vi "Query Output Operation Mode.vi"(8 "error in (no error)":errorcluster, 10 "Platform Slot Number (10)":i16=10 min=-1 max=255, 11 "VISA resource name":refnum<visa-resource-name>) -> (0 "error out":errorcluster, 2 "Operation Mode":string, 3 "VISA resource name out":refnum<visa-resource-name>)   [LabVIEW 2018, in "LTB-1.lvlib" / "3150.lvlib"]
doc: "Queries the current operation mode (ABSolute|XB|REFerence) for the active control mode (ATTenuation or POWer)."
uses:
  3150.lvlib
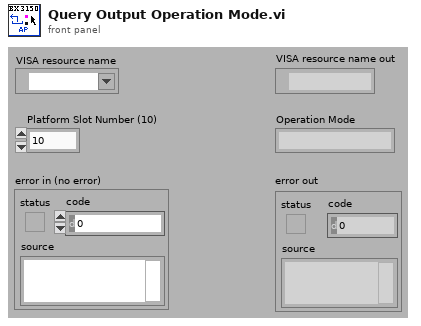
[diagram p1: front panel]
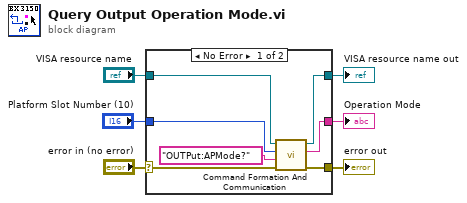
[diagram p0: block diagram]
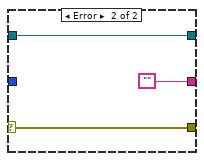
[diagram p2: hidden frame]
diagram:
  n1 = case shown="No Error" "error in (no error)" {
    selector: "error in (no error)" -> [w12 w15]
    tunnel: "VISA resource name" -> [w13 w16]
    tunnel: [w11 w16] -> w4
    tunnel: [w10 w15] -> w3
    tunnel: "Platform Slot Number (10)" -> [w8 _]
    tunnel: [w7 ""] -> w1
    frame No Error {
      n2 = call "Command Formation And Communication.vi"("error in (no error)"=w12, "Command"="OUTPut:APMode?", "Platform Slot Number"=w8, "VISA resource name"=w13) -> ("error out"=w10:errorcluster, "Response"=w7:string, "VISA resource name out"=w11:refnum<visa-resource-name>)  [unwired: 1 in, 4 out]
    }
    frame Error {
    }
  }
  "VISA resource name out" <- w4
  "error out" <- w3
  "Operation Mode" <- w1
